vi "Get I2C Channel Name.vi"(7 "I2C Channel Names":string[](array[string])=["A/I2C", "B/I2C"], 8 "Error In":errorcluster, 10 "I2C Channel":u8) -> (0 "Error Out":errorcluster, 2 "myRIO I2C Channels":string)   [LabVIEW 2011, in "LVH-LINX.lvlib" / "myRIO.lvlib"]
doc: "Get I2C channel names (strings) from channel numbers."
uses:
  myRIO.lvlib
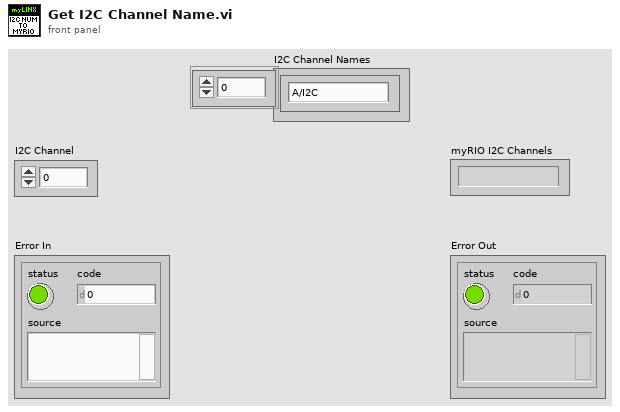
[diagram p1: front panel]
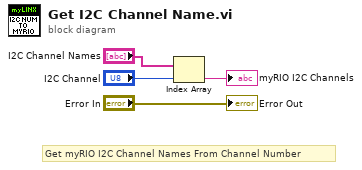
[diagram p0: block diagram]
diagram:
  # "Get myRIO I2C Channel Names From Channel Number"
  n1 = Index Array(array="I2C Channel Names", index="I2C Channel") -> (element=→"myRIO I2C Channels":string)
  "Error Out" <- "Error In"
